vi "Automatischer Ablauf Zustandsautomat.vi"(0 "Aktion":T1) -> (2 "Aktueller test":i32, 3 "Verwendete Spangaseingänge":i32[](array[numeric]), 4 "Aktion":T1, 6 "Anzeige aktualisieren":bool, 8 "Status":string)   [LabVIEW 2020, in "EPA 1065.lvlib" / "Gas Analyzer Drift 1065-550.lvlib"]
uses:
  Gas Analyzer Drift 1065-550.lvlib
  Aktion Automatischer Ablauf Zustandsautomat.ctl
  Seiten/CalGas Aufschaltung/FGV CalGas Aktionen.ctl
  Chiller NO2 1065-376/Aktion FGV Drift Daten.ctl
  Sprachverwaltung/FGV Aktion Tabelle zerlegen.ctl
  Allgemeine VIs/Aktion Test Status.ctl
  Funktionstasten/Zustaende.ctl
  Funktionstasten/Funktionstasten-Aktion.ctl
  Seiten/CalGas Aufschaltung/Auswahl Aufschaltpunkt.ctl
  PNS/Aktionen FGV Grenzwerte.ctl
  Seiten/FT-IR/FT-IR.lvlib
  Sprachverwaltung/Sprachverwaltung.lvlib
  Seiten/CalGas Aufschaltung/CalGas Aufschaltung.lvlib
  Funktionstasten/Funktionstasten.lvlib
  PNS/PNS.lvlib
  cRIO/PC/Kommunikation mit cRIO.lvlib
  Allgemein/allgemeine Sub-VIs.lvlib
  EPA 1065.lvlib
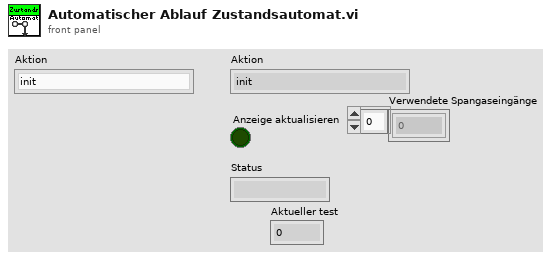
[diagram p1: front panel]
types:
  T1 = typedef "EPA 1065.lvlib/Gas Analyzer Drift 1065-550.lvlib/Aktion Automatischer Ablauf Zustandsautomat.ctl" = enum16{"init", "leerlauf", "N2 aufschalten", "N2 Aufschaltzeit warten", "N2 aufzeichnen", "CG aufschalten", "CG Aufschaltzeit warten", "CG aufzeichnen", "Span Auswahl ändern", "Test abgeschlossen", "Pre Test aktiv", "Post Test aktiv", "Störungen einlesen", "Störung", "Test anhalten", "Test fortsetzen", "Nachbehandlung init", "Nachbehandeln CG aufschalten", "Nachbehandeln CG warten", "Nachbehandeln CG aufzeichnen", "Abbrechen"}
  T2 = typedef "EPA 1065.lvlib/Aktion Test Status.ctl" = enum16{"init", "lesen", "prüfen", "Interference 366", "Interference 375", "Chiller läuft", "Drift läuft", "Pre Test läuft", "FID Optimization läuft", "FID Interference läuft"}
  T3 = typedef "EPA 1065.lvlib/Gas Analyzer Drift 1065-550.lvlib/Aktion FGV Drift Daten.ctl" = enum16{"lesen", "Konfig Daten", "PDF einstellen", "laden", "speichern", "Tabelle init", "Zeile Prüfen", "Info schreiben", "Span Einstellung", "Pre Werte schreiben", "Post Werte schreiben", "NB Pre Wert schreiben", "NB Post Wert schreiben", "Tabelle löschen"}
  T4 = typedef "Sprachverwaltung.lvlib/FGV Aktion Tabelle zerlegen.ctl" = enum16{"laden", "vereinzeln", "speichern"}
  T5 = typedef "CalGas Aufschaltung.lvlib/FGV CalGas Aktionen.ctl" = enum16{"lesen", "Analysator Auswahl", "Def.CalGas", "Aufschaltung CalGas", "laden", "speichern", "KAL extrahieren"}
  T6 = typedef "Funktionstasten.lvlib/Funktionstasten-Aktion.ctl" = enum16{"Initialisieren", "Zustand setzen", "Taste gedrückt", "Fehler speichern", "Lesen", "Manuell", "Remote", "Bitparallel", "Samplepoint", "Zeit Prüfen", "reset Umschalten"}
  T7 = typedef "Funktionstasten.lvlib/Zustaende.ctl" = enum16{"Standby", "Pause", "Eco", "Messen", "Kalibrieren", "Spülen Filter", "Spülen Leitung", "Umgebungsluft", "0-Gas", "Cal-Gas", "CG zu PNS", "-------------", "Init 1", "Init 2", "Init 3", "Init 4", "Messen vorbereiten", "Messen durchführen", "Exit"}
  T8 = typedef "CalGas Aufschaltung.lvlib/Auswahl Aufschaltpunkt.ctl" = enum16{"über Filterblock", "Analysator direkt", "über PNS", "Entnahme", "Gasdivider"}
  T9 = typedef "PNS.lvlib/Aktionen FGV Grenzwerte.ctl" = enum16{"lesen", "Grenzw. schreiben", "Anweisungscode", "IP-Adresse", "laden", "speichern", "Anweisungscode vorgeben"}
  T10 = cluster{"Pretest?":bool, "Spangaseingang":i32, "Tabellenbeginn":i32}
  T11 = cluster{"Pretest?":bool, "Spangaseingang":i32, "Tabellenbeginn":i32}[]
  T12 = typedef "CalGas Aufschaltung.lvlib/Aufschaltung CalGas.ctl" = cluster{"Kalibriergas":T13, "Aufschaltpunkt":T8, "Analysator":T14}
  T13 = typedef "Auswahlfeld.ctl" = u16
  T14 = typedef "CalGas Aufschaltung.lvlib/Auswahl Analysator.ctl" = enum16{"FT-IR", "FID", "PMA", "PMA/FID/FT-IR"}
  T15 = typedef "EPA 1065.lvlib/Gas Analyzer Drift 1065-550.lvlib/Spaninlet Cluster.ctl" = cluster{"Span Inlet Active":T16, "Analysator":T17, "Konfig Gasflasche":T16, "Gasflasche":T18, "Gasflaschen Nr.:":string, "Ablaufdatum":timestamp, "Modus":T19, "Komponenten":T20}
  T16 = typedef "System Einstellungen V2.lvlib/Konfig Gasflasche.ctl" = bool
  T17 = typedef "System Einstellungen V2.lvlib/Analysatoren.ctl" = string
  T18 = typedef "System Einstellungen V2.lvlib/Gasflasche Auswahl.ctl" = u16
  T19 = typedef "EPA 1065.lvlib/T90 Test 1065-308.lvlib/Modus.ctl" = u16
  T20 = typedef "EPA 1065.lvlib/Gas Analyzer Drift 1065-550.lvlib/Komponentencluster.ctl" = cluster{"Komponente 1":T21, "Komponente 2":T21, "Komponente 3":T21, "Komponente 4":T21, "Komponente 5":T21}
  T21 = typedef "EPA 1065.lvlib/Gas Analyzer Drift 1065-550.lvlib/Komponentenauswahl.ctl" = cluster{"Komponente:":u16, "Konzentration IST":dbl, "Einheit":enum16{"ppm", "%"}, "Genauigkeit":dbl}
  T22 = typedef "EPA 1065.lvlib/Gas Analyzer Drift 1065-550.lvlib/Konfig Daten Drift Verification.ctl" = cluster{"Bearbeiter:":string, "Pfad:":path, "Textname:":string, "CG Aufschaltzeit:":dbl, "N2 Aufschaltzeit:":dbl}
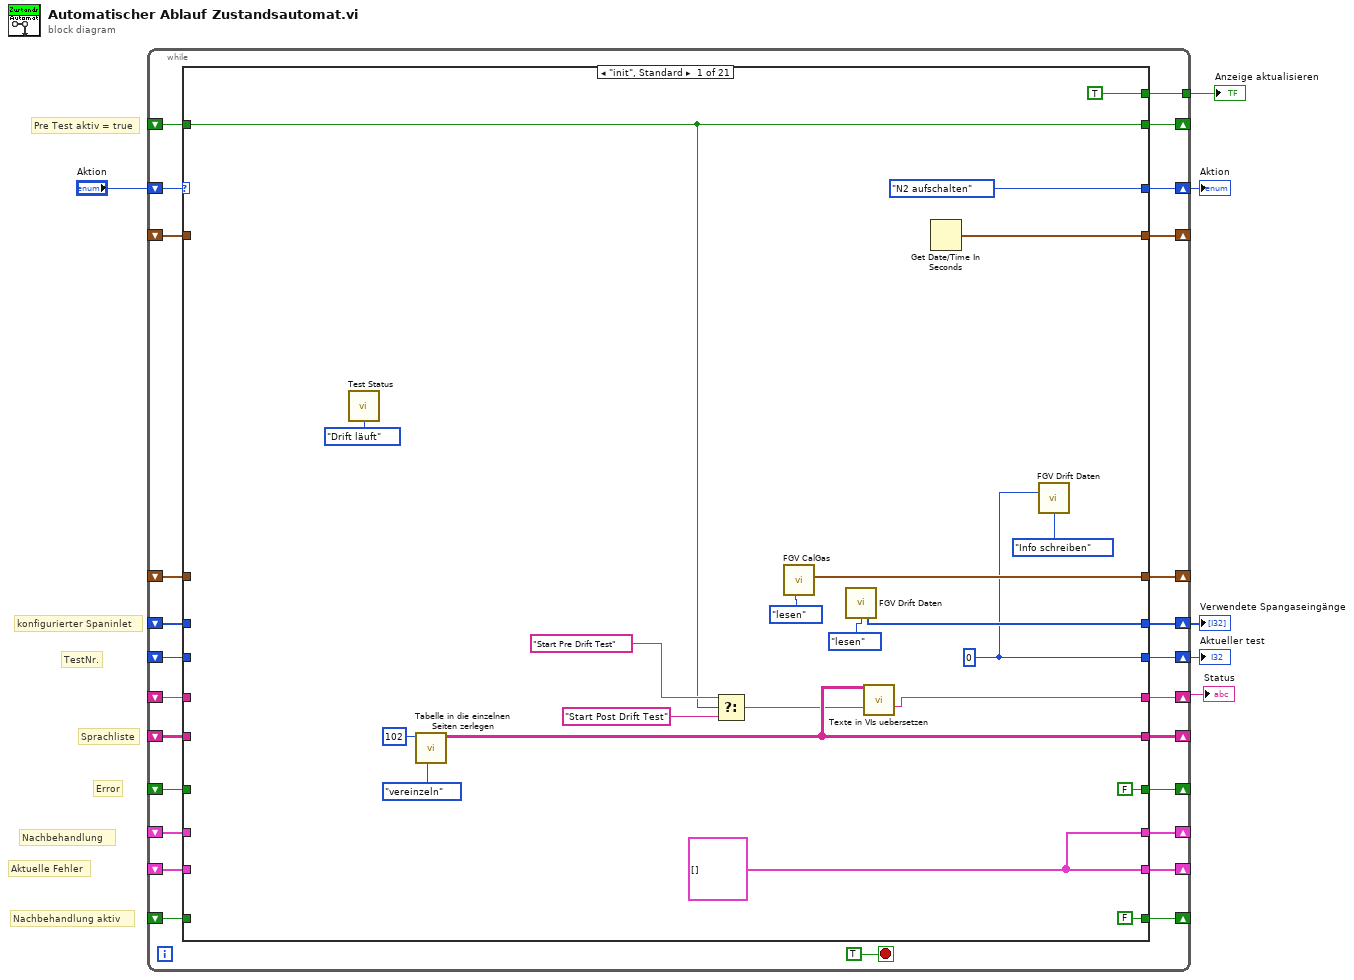
[diagram p0: block diagram]
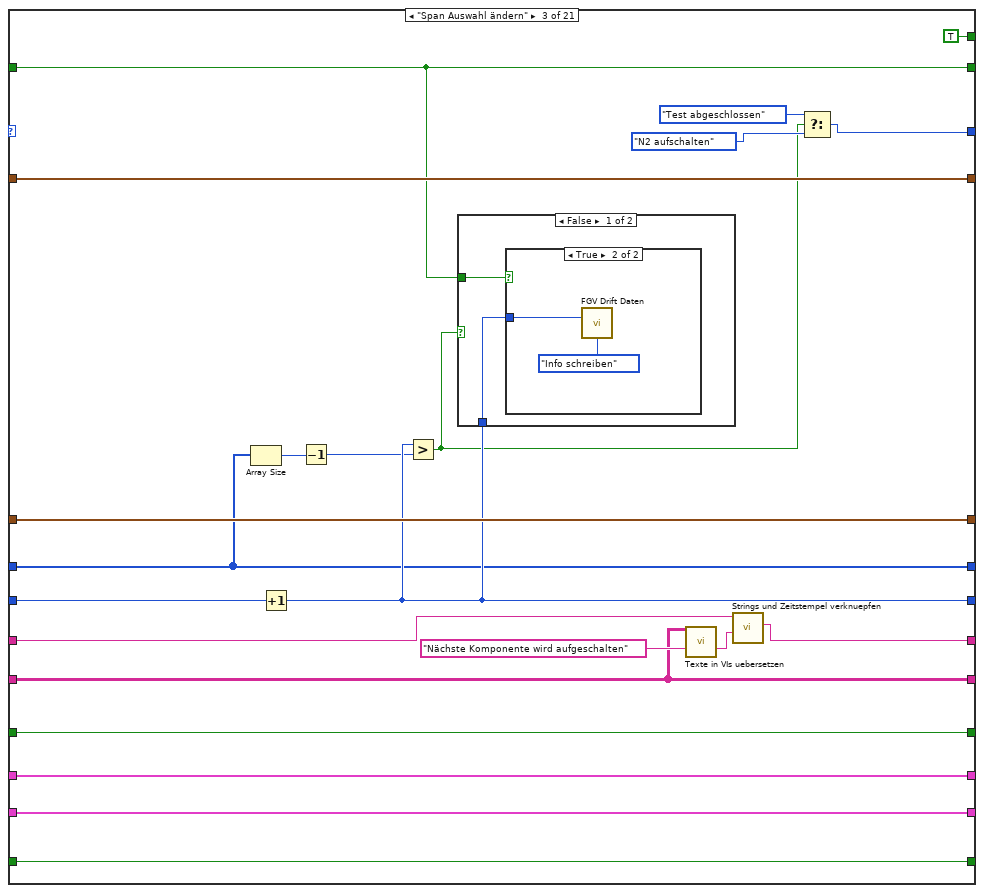
[diagram p3: hidden frame]
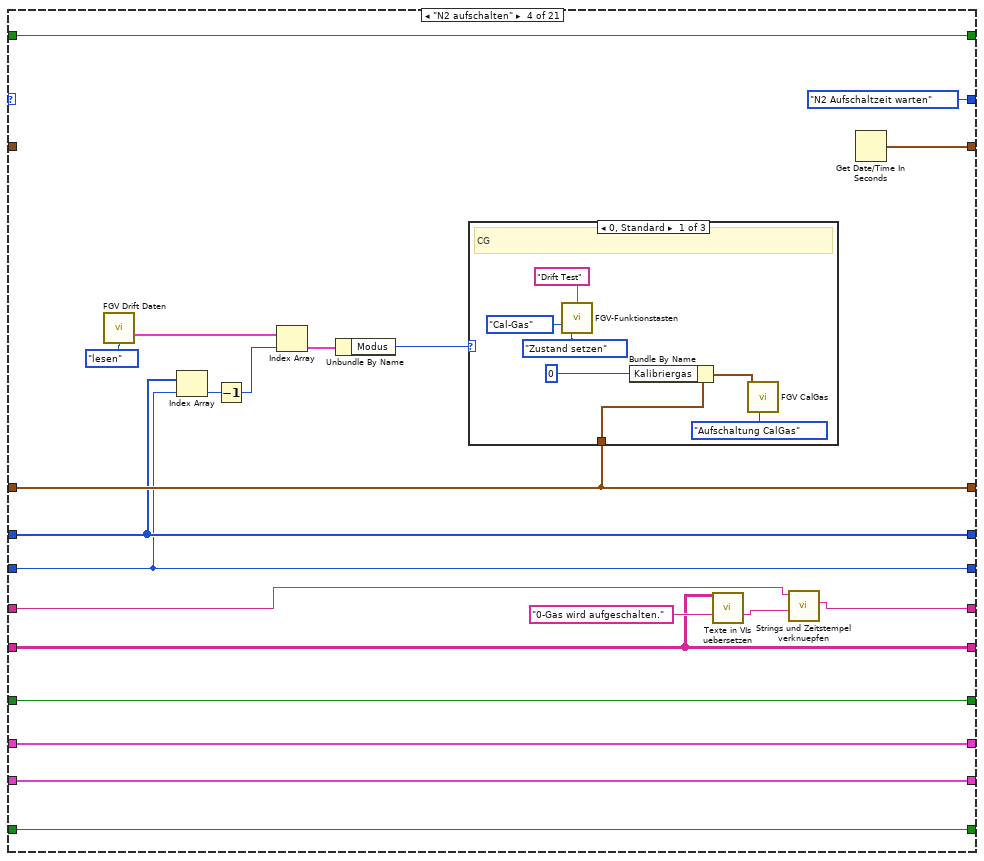
[diagram p6: hidden frame]
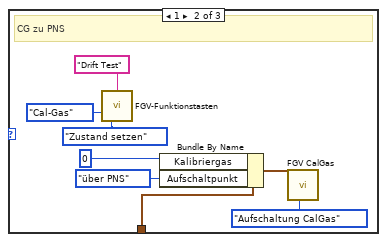
[diagram p7: hidden frame]
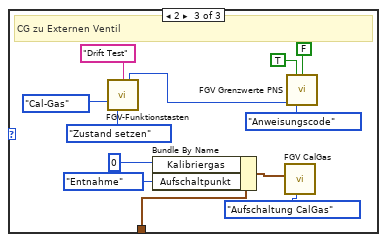
[diagram p8: hidden frame]
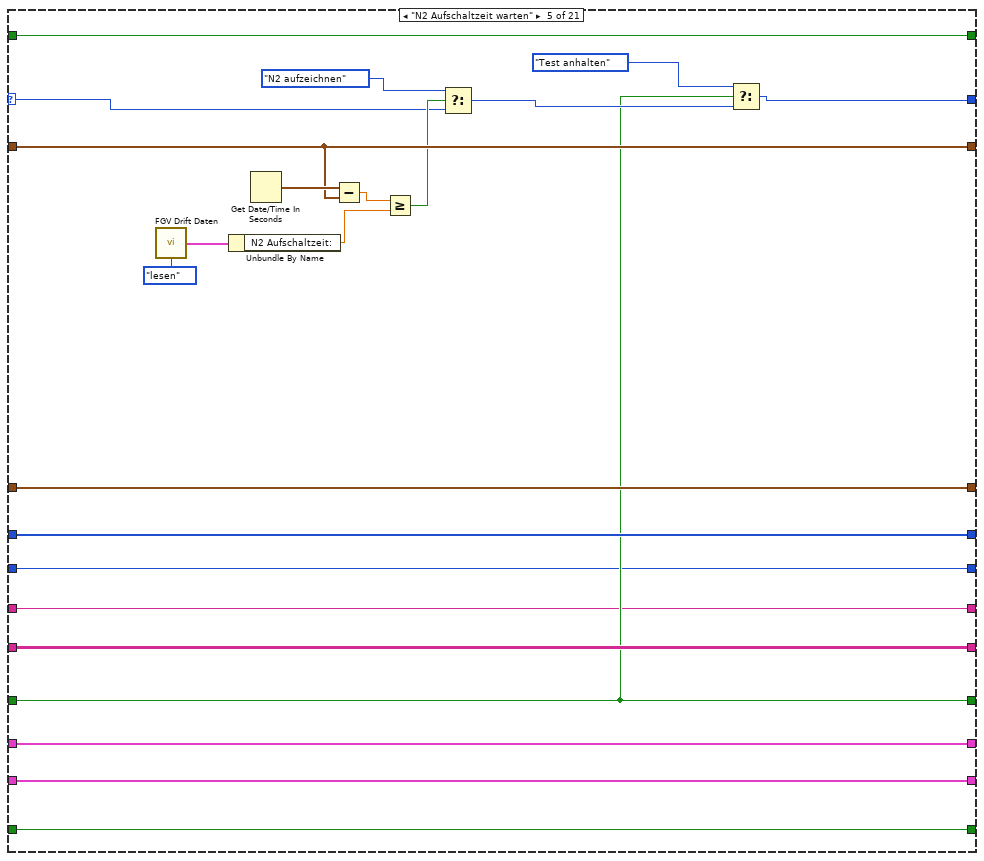
[diagram p9: hidden frame]
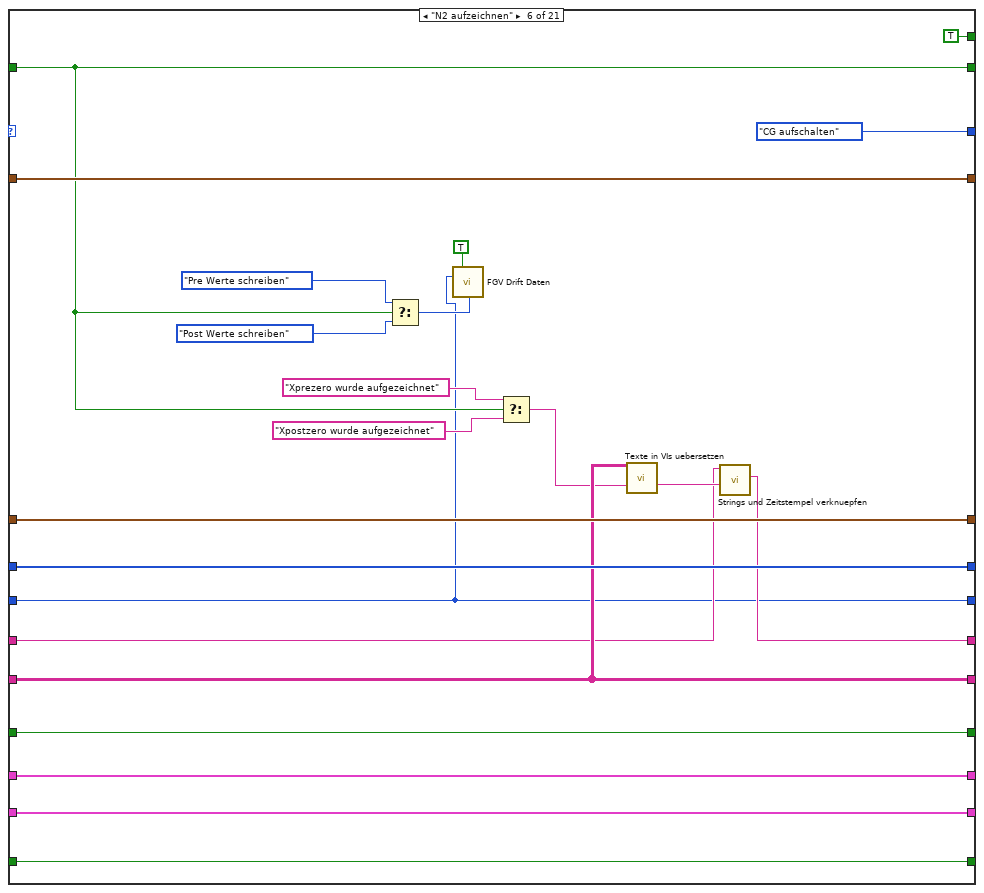
[diagram p10: hidden frame]
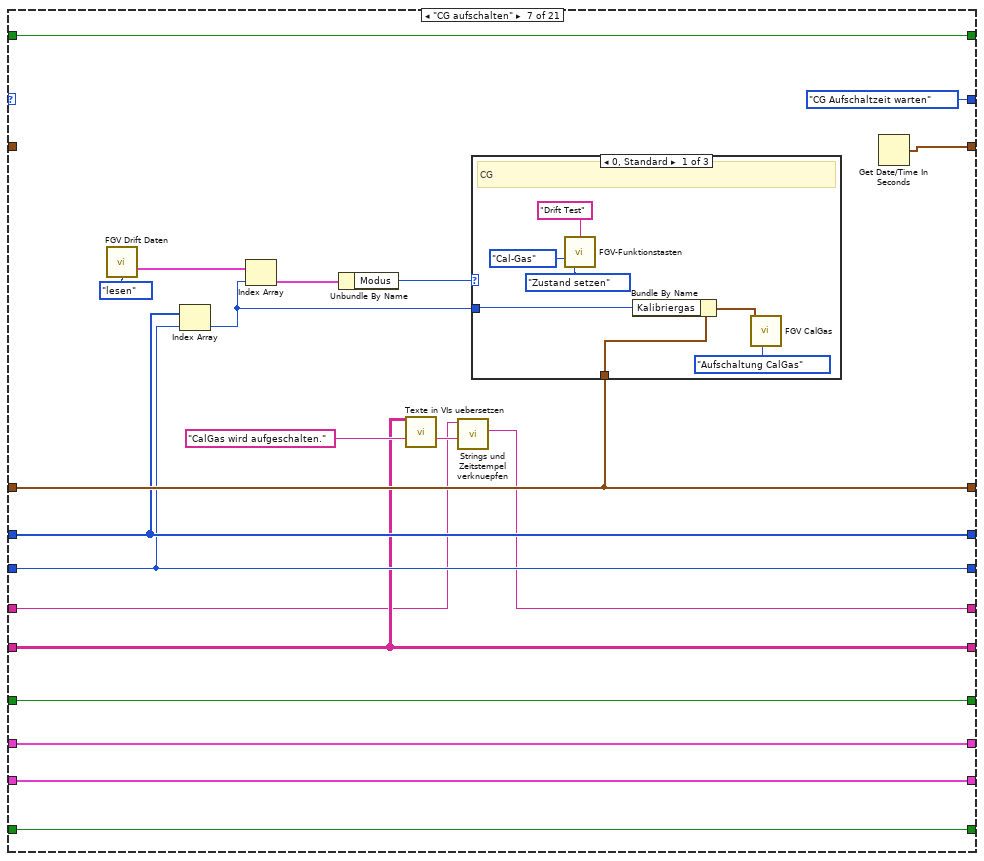
[diagram p11: hidden frame]
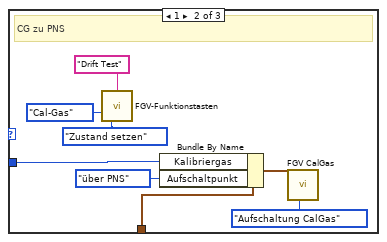
[diagram p12: hidden frame]
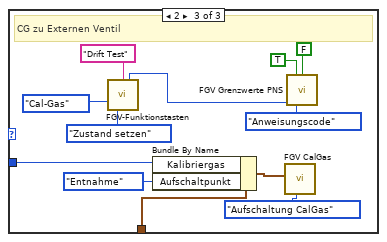
[diagram p13: hidden frame]
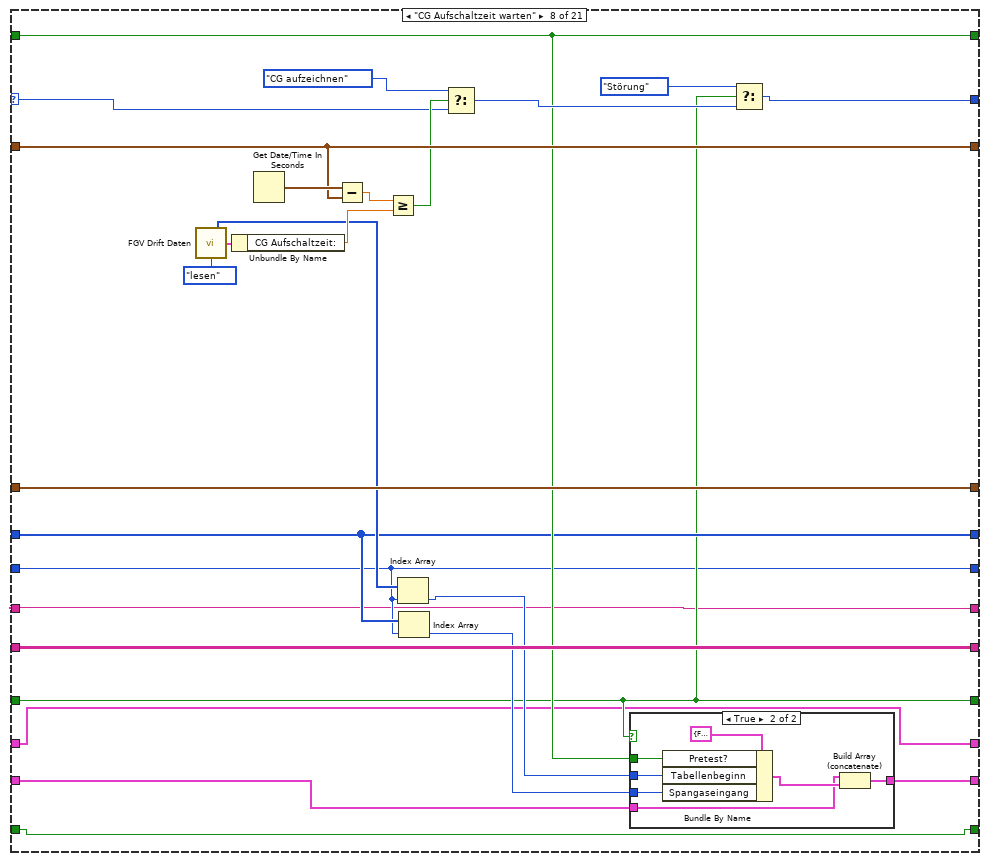
[diagram p14: hidden frame]
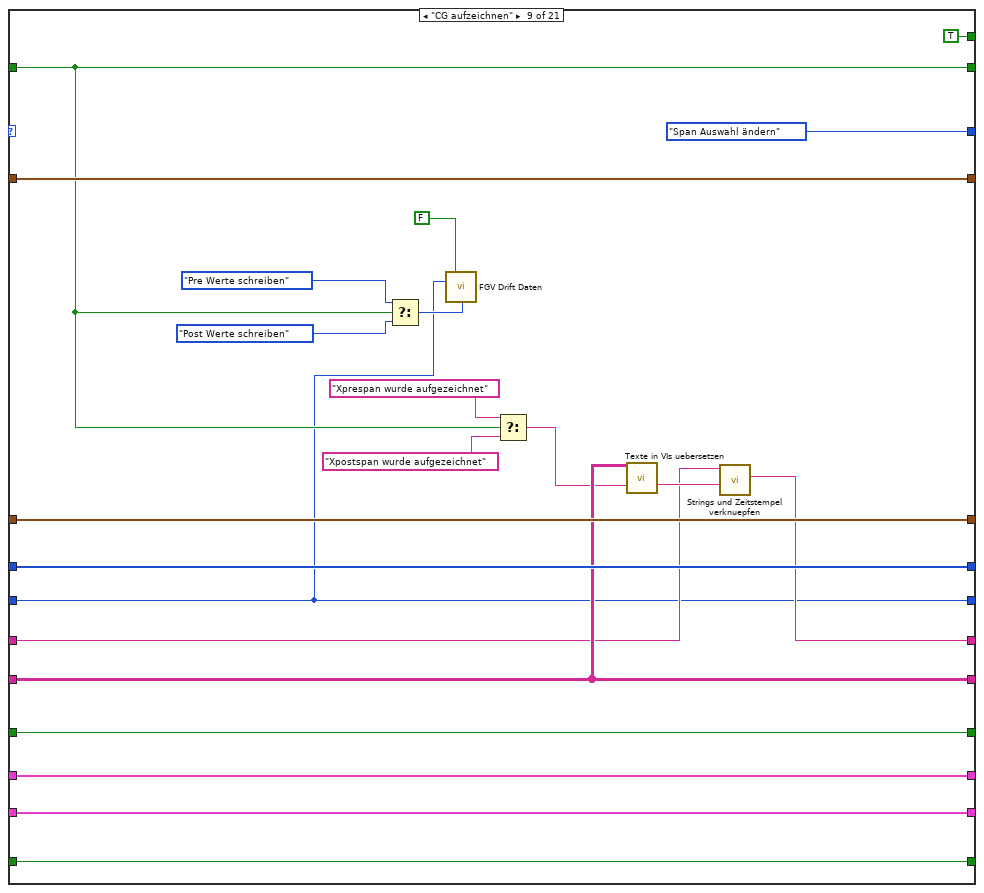
[diagram p16: hidden frame]
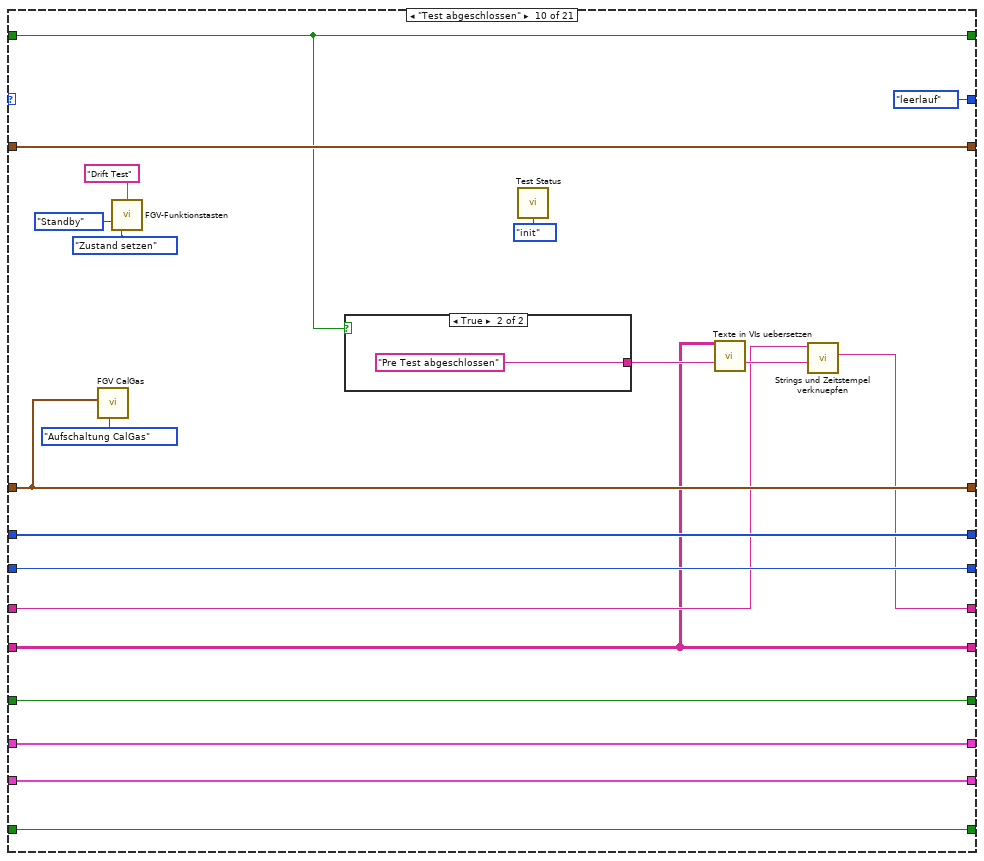
[diagram p17: hidden frame]
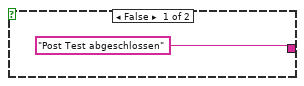
[diagram p18: hidden frame]
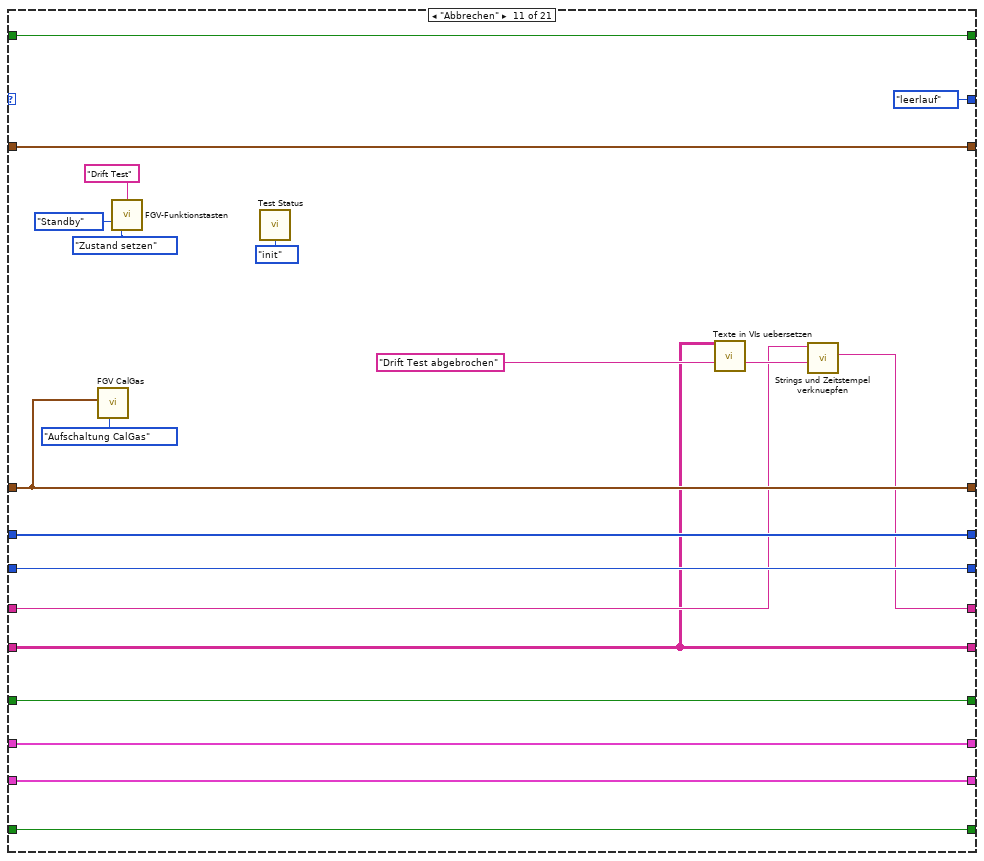
[diagram p19: hidden frame]
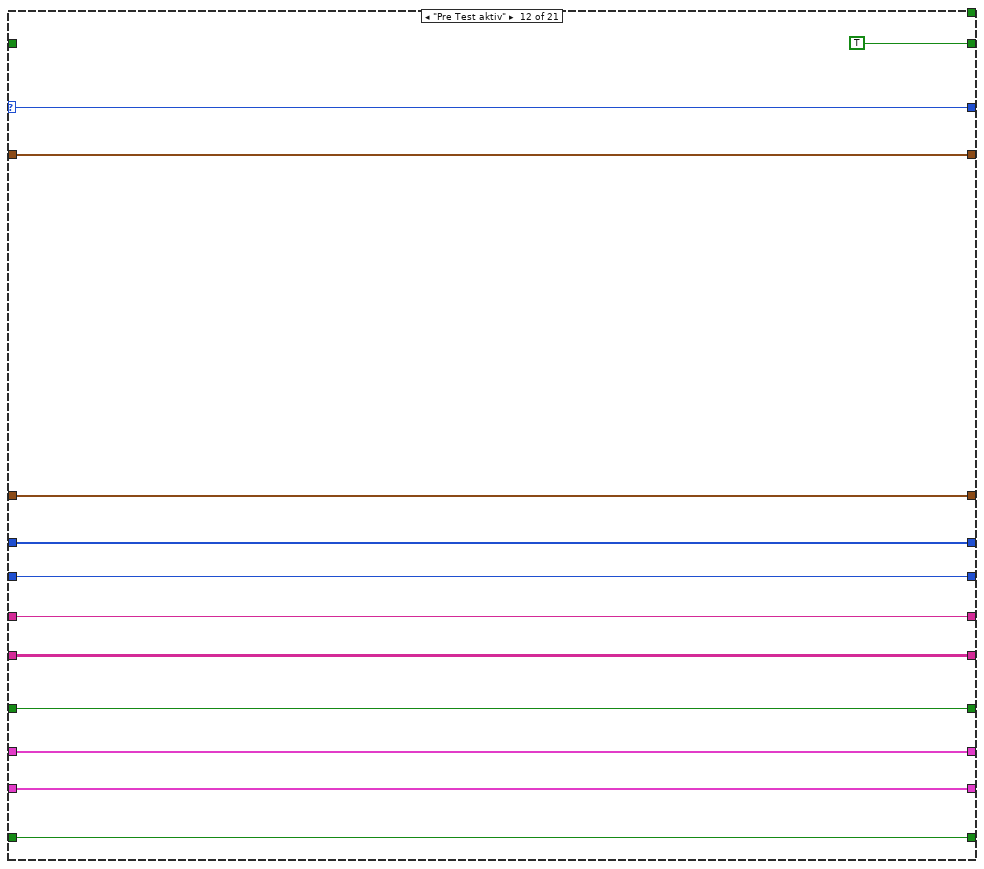
[diagram p20: hidden frame]
diagram:
  # "Nachbehandlung"
  # "Aktuelle Fehler"
  # "Nachbehandlung aktiv"
  # "TestNr."
  # "Sprachliste"
  # "Error"
  # "konfigurierter Spaninlet"
  # "Pre Test aktiv = true"
  n1 = while {
    shift-right: [w30] -> w1
    shift-left: _ -> [w29]
    shift-right: [w27] -> _
    shift-left: _ -> [w26]
    shift-right: [w25] -> _
    shift-left: _ -> [w24]
    shift-right: [w23] -> w4
    shift-left: "Aktion" -> [w31]
    shift-right: [w28] -> w2
    shift-left: _ -> [w22]
    shift-right: [w21] -> w3
    shift-left: _ -> [w20]
    shift-right: [w19] -> _
    shift-left: _ -> [w18]
    shift-right: [w17] -> _
    shift-left: _ -> [w16]
    shift-right: [w15] -> _
    shift-left: _ -> [w14]
    shift-right: [w13] -> _
    shift-left: _ -> [w12]
    shift-right: [w11] -> _
    shift-left: _ -> [w10]
    shift-right: [w9] -> _
    shift-left: _ -> [w8]
    tunnel: [w7] -> w5
    stop <- TRUE stop-if-true
    n2 = case shown="\"init\", Standard" w31 {
      selector: w31 -> [_ w54 _ _ w153 _ _ w248 _ _ _ w336 w349 w360 _ _ _ _ _ w507 _]
      tunnel: [w39 w59 w67 w94 w140 w175 w188 w231 w276 w289 w311 w334 w341 w358 w380 w402 w416 w427 w451 w492 w531] -> w30
      tunnel: w29 -> [_ w59 w68 w95 w140 w176 w189 w231 w277 w291 w313 w334 w341 w358 w381 w403 w417 w428 w452 w492 w532]
      tunnel: [w44 w57 w82 w106 w143 w167 w197 w234 w269 w302 w324 w335 w344 w359 w386 w400 w415 0 w449 w494 w523] -> w28
      tunnel: [w34 w65 w83 w112 w147 w173 w203 w242 w274 w288 w310 TRUE FALSE w377 w392 w411 w426 w431 w446 w501 w529] -> w27
      tunnel: w26 -> [w34 w65 w83 w112 w147 w173 w203 w242 w274 w288 w310 _ _ w377 w392 w411 w426 w431 _ w501 w529]
      tunnel: [w52 w64 w87 w111 w161 w183 w202 w256 w286 w299 w321 w339 w351 w376 w391 w394 w425 w436 w464 w515 w541] -> w25
      tunnel: w24 -> [_ w64 w87 w111 w161 w183 w202 w256 w286 w299 w321 w339 w351 w376 w391 w394 w425 w436 w464 w515 w541]
      tunnel: [Aktion_Automatischer_Ablauf_Zustandsautomat."N2 aufschalten" ("Aktion") w54 w77 Aktion_Automatischer_Ablauf_Zustandsautomat."N2 Aufschaltzeit warten" ("Aktion") w148 Aktion_Automatischer_Ablauf_Zustandsautomat."CG aufschalten" ("Aktion") Aktion_Automatischer_Ablauf_Zustandsautomat."CG Aufschaltzeit warten" ("Aktion") w243 Aktion_Automatischer_Ablauf_Zustandsautomat."Span Auswahl ändern" ("Aktion") Aktion_Automatischer_Ablauf_Zustandsautomat."leerlauf" ("Aktion") Aktion_Automatischer_Ablauf_Zustandsautomat."leerlauf" ("Aktion") w336 w349 w360 Aktion_Automatischer_Ablauf_Zustandsautomat."Span Auswahl ändern" ("Aktion") Aktion_Automatischer_Ablauf_Zustandsautomat."leerlauf" ("Aktion") Aktion_Automatischer_Ablauf_Zustandsautomat."N2 aufschalten" ("Aktion") Aktion_Automatischer_Ablauf_Zustandsautomat."Nachbehandeln CG aufschalten" ("Aktion") Aktion_Automatischer_Ablauf_Zustandsautomat."Nachbehandeln CG warten" ("Aktion") w502 Aktion_Automatischer_Ablauf_Zustandsautomat."Span Auswahl ändern" ("Aktion")] -> w23
      tunnel: w22 -> [_ w57 w84 w106 w143 w167 w197 w234 w269 w302 w324 w335 w344 w359 w386 w400 w415 _ w449 w494 w523]
      tunnel: [w49 w63 w81 w107 w146 w182 w198 w240 w285 w306 w328 w338 w350 w375 w390 w410 w424 w438 w460 w500 w540] -> w21
      tunnel: w20 -> [_ w63 w81 w107 w146 w182 w198 w240 w285 w306 w328 w338 w350 w375 w390 w410 w424 w438 w460 w500 w540]
      tunnel: [FALSE w62 w86 w103 w145 w181 w194 w235 w284 w305 w327 w337 w348 w362 w389 w409 w423 FALSE w458 w497 w539] -> w19
      tunnel: w18 -> [_ w62 w86 w103 w145 w181 w194 w235 w284 w305 w327 w337 w348 _ w389 w409 w423 _ w458 w497 w539]
      tunnel: [w47 w61 w85 w99 w155 w180 w184 w250 w283 w304 w326 w333 w347 w357 w388 w408 w422 w441 w457 w509 w538] -> w17
      tunnel: w16 -> [_ w61 w85 _ w155 w180 _ w250 w283 w304 w326 w333 w347 w357 w388 w408 w422 _ w457 w509 w538]
      tunnel: [w40 w60 w69 w96 w151 w178 w190 w246 w279 w290 w312 w332 w346 w356 w378 w404 w418 w430 w453 w505 w534] -> w15
      tunnel: w14 -> [_ w60 w69 w96 w151 w178 w190 w246 w279 w290 w312 w332 w346 w356 w378 w404 w418 w430 w453 w505 w534]
      tunnel: [w41 w58 w74 w102 w144 w165 w187 w237 w268 w303 w325 w331 w345 w355 w387 w407 w421 w439 w448 w499 w522] -> w13
      tunnel: w12 -> [_ w58 w74 w102 w144 w165 w187 w236 w268 w303 w325 w331 w345 w355 w387 w407 w421 w439 w448 w498 w522]
      tunnel: [FALSE w56 w73 w101 w142 w164 w186 w233 w267 w301 w323 w330 w343 w354 w385 w396 w413 TRUE w450 w496 w524] -> w11
      tunnel: w10 -> [_ w56 w73 w101 w142 w164 w186 w233 w267 w301 w323 w330 w343 w354 w385 w396 w413 _ w450 w496 w524]
      tunnel: [w41 w55 w72 w100 w141 w163 w185 w232 w266 w294 w316 w329 w342 w353 w384 w393 w412 w435 w444 w495 w521] -> w9
      tunnel: w8 -> [_ w55 w72 w100 w141 w163 w185 w232 w266 w294 w316 w329 w342 w353 w384 w393 w412 w435 w444 w495 w521]
      tunnel: [TRUE _ TRUE _ _ TRUE _ _ TRUE _ _ _ _ _ _ _ _ _ _ _ TRUE] -> w7
      frame "init", Default {
        w41 = T11 []
        w44 = 0
        n3 = call "Test Status.vi"("Aktion"=Aktion_Test_Status."Drift läuft") -> ()  [unwired: 11 in, 4 out]
        n4 = call "Tabelle in die einzelnen Seiten zerlegen.vi"("Aktion"=FGV_Aktion_Tabelle_zerlegen."vereinzeln", "Index (Seite)"=102) -> ("Sprachliste"=w40:string[][])  [unwired: 7 in, 2 out]
        n5 = Select(t="Start Pre Drift Test", s=w34, f="Start Post Drift Test") -> (s? t:f=w33:string)
        n6 = call "FGV CalGas.vi"("Aktionen"=FGV_CalGas_Aktionen."lesen") -> ("Aufschaltung CalGas"=w52:T12)  [unwired: 6 in, 4 out]
        n7 = call "FGV Drift Daten.vi"("Aktion"=Aktion_FGV_Drift_Daten."lesen") -> ("Verwendete Spangaseingänge"=w49:i32[])  [unwired: 7 in, 7 out]
        n8 = call "Texte in VIs uebersetzen.vi"("Sprachliste"=w40, "String zum Übersetzen"=w33) -> ("String zum Übersetzen"=w39:string)  [unwired: 9 in, 4 out]
        n9 = Get Date/Time In Seconds() -> (seconds since 1Jan1904=w47:timestamp)
        n10 = call "FGV Drift Daten.vi"("Testnr."=w44, "Aktion"=Aktion_FGV_Drift_Daten."Info schreiben") -> ()  [unwired: 6 in, 8 out]
      }
      frame "leerlauf" {
      }
      frame "Span Auswahl ändern" {
        n11 = Array Size(array=w81) -> (size(s)=w80:i32)
        n12 = Increment(x=w84) -> (x+1=w82:i32)
        n13 = Decrement(x=w80) -> (x-1=w79:i32)
        n14 = Greater?(x=w82, y=w79) -> (0:w75:bool)
        n15 = case shown="False" w75 {
          tunnel: w83 -> [w89 _]
          tunnel: w82 -> [w88 _]
          frame False {
            n16 = case shown="True" w89 {
              tunnel: w88 -> [_ w90]
              frame False {
              }
              frame True {
                n17 = call "FGV Drift Daten.vi"("Testnr."=w90, "Aktion"=Aktion_FGV_Drift_Daten."Info schreiben") -> ()  [unwired: 6 in, 8 out]
              }
            }
          }
          frame True {
          }
        }
        n18 = call "Texte in VIs uebersetzen.vi"("Sprachliste"=w69, "String zum Übersetzen"="Nächste Komponente wird aufgeschalten" ("String 1 hinzufügen")) -> ("String zum Übersetzen"=w71:string)  [unwired: 9 in, 4 out]
        n19 = call "Strings und Zeitstempel verknuepfen.vi"("String 1 hinzufügen"=w71, "Eingagns String"=w68) -> ("Verknüpfter String"=w67:string)  [unwired: 9 in]
        n20 = Select(t=Aktion_Automatischer_Ablauf_Zustandsautomat."Test abgeschlossen", s=w75, f=Aktion_Automatischer_Ablauf_Zustandsautomat."N2 aufschalten" ("Aktion")) -> (s? t:f=w77:T1)
      }
      frame "N2 aufschalten" {
        n21 = call "FGV Drift Daten.vi"("Aktion"=Aktion_FGV_Drift_Daten."lesen") -> ("Spangaseinstellungen"=w109:T15[])  [unwired: 7 in, 7 out]
        n22 = Index Array(array=w107, index=w106) -> (element=w105:i32)
        n23 = Decrement(x=w105) -> (x-1=w92:i32)
        n24 = Index Array(array=w109, index=w92) -> (element=w108:T15)
        n25 = Unbundle By Name(w108) -> ("Modus"=w104:T19)
        n26 = case shown="0, Standard" w104 {
          tunnel: w111 -> [w114 w121 w129]
          frame 0, Default {
            # "CG"
            n27 = call "FGV-Funktionstasten.vi"("Herkunft"="Drift Test", "Zustand"=Zustaende."Cal-Gas", "Aktion"=Funktionstasten-Aktion."Zustand setzen") -> ()  [unwired: 5 in, 8 out]
            n28 = Bundle By Name(cluster=w114, "Kalibriergas"=u16 0) -> (w115:T12)
            n29 = call "FGV CalGas.vi"("Aktionen"=FGV_CalGas_Aktionen."Aufschaltung CalGas", "Aufschaltung CalGas"=w115) -> ()  [unwired: 5 in, 5 out]
          }
          frame 1 {
            # "CG zu PNS"
            n30 = call "FGV-Funktionstasten.vi"("Herkunft"="Drift Test", "Zustand"=Zustaende."Cal-Gas", "Aktion"=Funktionstasten-Aktion."Zustand setzen") -> ()  [unwired: 5 in, 8 out]
            n31 = Bundle By Name(cluster=w121, "Kalibriergas"=u16 0, "Aufschaltpunkt"=Auswahl_Aufschaltpunkt."über PNS") -> (w122:T12)
            n32 = call "FGV CalGas.vi"("Aktionen"=FGV_CalGas_Aktionen."Aufschaltung CalGas", "Aufschaltung CalGas"=w122) -> ()  [unwired: 5 in, 5 out]
          }
          frame 2 {
            # "CG zu Externen Ventil"
            n33 = call "FGV-Funktionstasten.vi"("Herkunft"="Drift Test", "Zustand"=Zustaende."Cal-Gas", "Aktion"=Funktionstasten-Aktion."Zustand setzen") -> ("Samplepoint"=w133:u16)  [unwired: 5 in, 7 out]
            n34 = Bundle By Name(cluster=w129, "Kalibriergas"=u16 0, "Aufschaltpunkt"=Auswahl_Aufschaltpunkt."Entnahme") -> (w130:T12)
            n35 = call "FGV CalGas.vi"("Aktionen"=FGV_CalGas_Aktionen."Aufschaltung CalGas", "Aufschaltung CalGas"=w130) -> ()  [unwired: 5 in, 5 out]
            n36 = call "FGV Grenzwerte PNS.vi"("T90"=TRUE ("T90 lüften"), "T90 lüften"=FALSE, "Samplepoint"=w133, "Aktionen FGV Grenzwerte"=Aktionen_FGV_Grenzwerte."Anweisungscode") -> ()  [unwired: 9 in, 3 out]
          }
        }
        n37 = call "Texte in VIs uebersetzen.vi"("Sprachliste"=w96, "String zum Übersetzen"="0-Gas wird aufgeschalten." ("String 1 hinzufügen")) -> ("String zum Übersetzen"=w93:string)  [unwired: 9 in, 4 out]
        n38 = call "Strings und Zeitstempel verknuepfen.vi"("String 1 hinzufügen"=w93, "Eingagns String"=w95) -> ("Verknüpfter String"=w94:string)  [unwired: 9 in]
        n39 = Get Date/Time In Seconds() -> (seconds since 1Jan1904=w99:timestamp)
      }
      frame "N2 Aufschaltzeit warten" {
        n40 = call "FGV Drift Daten.vi"("Aktion"=Aktion_FGV_Drift_Daten."lesen") -> ("Drift Konfig Daten"=w159:T22)  [unwired: 7 in, 7 out]
        n41 = Unbundle By Name(w159) -> ("N2 Aufschaltzeit:"=w157:dbl)
        n42 = Get Date/Time In Seconds() -> (seconds since 1Jan1904=w160:timestamp)
        n43 = Subtract(x=w160, y=w155) -> (x-y=w158:dbl)
        n44 = Greater Or Equal?(x=w158, y=w157) -> (x >= y?=w154:bool)
        n45 = Select(t=Aktion_Automatischer_Ablauf_Zustandsautomat."N2 aufzeichnen", s=w154, f=w153) -> (s? t:f=w149:T1)
        n46 = Select(t=Aktion_Automatischer_Ablauf_Zustandsautomat."Test anhalten", s=w145, f=w149) -> (s? t:f=w148:T1)
      }
      frame "N2 aufzeichnen" {
        n47 = Select(t=Aktion_FGV_Drift_Daten."Pre Werte schreiben" ("Aktion"), s=w173, f=Aktion_FGV_Drift_Daten."Post Werte schreiben" ("Aktion")) -> (s? t:f=w171:T3)
        n48 = call "FGV Drift Daten.vi"("0-Gas Wert?"=TRUE, "Testnr."=w167, "Aktion"=w171) -> ()  [unwired: 5 in, 8 out]
        n49 = Select(t="Xprezero wurde aufgezeichnet" ("String 1 hinzufügen"), s=w173, f="Xpostzero wurde aufgezeichnet" ("String 1 hinzufügen")) -> (s? t:f=w177:string)
        n50 = call "Texte in VIs uebersetzen.vi"("Sprachliste"=w178, "String zum Übersetzen"=w177) -> ("String zum Übersetzen"=w179:string)  [unwired: 9 in, 4 out]
        n51 = call "Strings und Zeitstempel verknuepfen.vi"("String 1 hinzufügen"=w179, "Eingagns String"=w176) -> ("Verknüpfter String"=w175:string)  [unwired: 9 in]
      }
      frame "CG aufschalten" {
        n52 = call "FGV Drift Daten.vi"("Aktion"=Aktion_FGV_Drift_Daten."lesen") -> ("Spangaseinstellungen"=w200:T15[])  [unwired: 7 in, 7 out]
        n53 = Index Array(array=w198, index=w197) -> (element=w195:i32)
        n54 = Index Array(array=w200, index=w195) -> (element=w199:T15)
        n55 = Unbundle By Name(w199) -> ("Modus"=w196:T19)
        n56 = call "Texte in VIs uebersetzen.vi"("Sprachliste"=w190, "String zum Übersetzen"="CalGas wird aufgeschalten." ("String 1 hinzufügen")) -> ("String zum Übersetzen"=w192:string)  [unwired: 9 in, 4 out]
        n57 = call "Strings und Zeitstempel verknuepfen.vi"("String 1 hinzufügen"=w192, "Eingagns String"=w189) -> ("Verknüpfter String"=w188:string)  [unwired: 9 in]
        n58 = case shown="0, Standard" w196 {
          tunnel: w202 -> [w205 w212 w220]
          tunnel: w195 -> [w204 w211 w219]
          frame 0, Default {
            # "CG"
            n59 = call "FGV-Funktionstasten.vi"("Herkunft"="Drift Test", "Zustand"=Zustaende."Cal-Gas", "Aktion"=Funktionstasten-Aktion."Zustand setzen") -> ()  [unwired: 5 in, 8 out]
            n60 = Bundle By Name(cluster=w205, "Kalibriergas"=w204) -> (w206:T12)
            n61 = call "FGV CalGas.vi"("Aktionen"=FGV_CalGas_Aktionen."Aufschaltung CalGas", "Aufschaltung CalGas"=w206) -> ()  [unwired: 5 in, 5 out]
          }
          frame 1 {
            # "CG zu PNS"
            n62 = call "FGV-Funktionstasten.vi"("Herkunft"="Drift Test", "Zustand"=Zustaende."Cal-Gas", "Aktion"=Funktionstasten-Aktion."Zustand setzen") -> ()  [unwired: 5 in, 8 out]
            n63 = Bundle By Name(cluster=w212, "Kalibriergas"=w211, "Aufschaltpunkt"=Auswahl_Aufschaltpunkt."über PNS") -> (w213:T12)
            n64 = call "FGV CalGas.vi"("Aktionen"=FGV_CalGas_Aktionen."Aufschaltung CalGas", "Aufschaltung CalGas"=w213) -> ()  [unwired: 5 in, 5 out]
          }
          frame 2 {
            # "CG zu Externen Ventil"
            n65 = call "FGV-Funktionstasten.vi"("Herkunft"="Drift Test", "Zustand"=Zustaende."Cal-Gas", "Aktion"=Funktionstasten-Aktion."Zustand setzen") -> ("Samplepoint"=w224:u16)  [unwired: 5 in, 7 out]
            n66 = Bundle By Name(cluster=w220, "Kalibriergas"=w219, "Aufschaltpunkt"=Auswahl_Aufschaltpunkt."Entnahme") -> (w221:T12)
            n67 = call "FGV CalGas.vi"("Aktionen"=FGV_CalGas_Aktionen."Aufschaltung CalGas", "Aufschaltung CalGas"=w221) -> ()  [unwired: 5 in, 5 out]
            n68 = call "FGV Grenzwerte PNS.vi"("T90"=TRUE ("T90 lüften"), "T90 lüften"=FALSE, "Samplepoint"=w224, "Aktionen FGV Grenzwerte"=Aktionen_FGV_Grenzwerte."Anweisungscode") -> ()  [unwired: 9 in, 3 out]
          }
        }
        n69 = Get Date/Time In Seconds() -> (seconds since 1Jan1904=w184:timestamp)
      }
      frame "CG Aufschaltzeit warten" {
        n70 = call "FGV Drift Daten.vi"("Aktion"=Aktion_FGV_Drift_Daten."lesen") -> ("Tabellenbeginn"=w241:i32[], "Drift Konfig Daten"=w254:T22)  [unwired: 7 in, 6 out]
        n71 = Unbundle By Name(w254) -> ("CG Aufschaltzeit:"=w252:dbl)
        n72 = Get Date/Time In Seconds() -> (seconds since 1Jan1904=w255:timestamp)
        n73 = Subtract(x=w255, y=w250) -> (x-y=w253:dbl)
        n74 = Greater Or Equal?(x=w253, y=w252) -> (x >= y?=w249:bool)
        n75 = Index Array(array=w241, index=w234) -> (element=w239:i32)
        n76 = Index Array(array=w240, index=w234) -> (element=w238:i32)
        n77 = Select(t=Aktion_Automatischer_Ablauf_Zustandsautomat."CG aufzeichnen", s=w249, f=w248) -> (s? t:f=w244:T1)
        n78 = case shown="True" w235 {
          tunnel: w242 -> [_ w264]
          tunnel: w239 -> [_ w262]
          tunnel: w238 -> [_ w261]
          tunnel: [w257 w259] -> w237
          tunnel: w236 -> [w257 w258]
          frame False {
          }
          frame True {
            n79 = Bundle By Name(cluster=T10 {"Pretest?"=FALSE, "Spangaseingang"=0, "Tabellenbeginn"=0} ("Eingangs-Cluster"), "Pretest?"=w264, "Tabellenbeginn"=w262, "Spangaseingang"=w261) -> (w260:T10)
            n80 = Build Array (concatenate)(w258, w260) -> (w259:T11)
          }
        }
        n81 = Select(t=Aktion_Automatischer_Ablauf_Zustandsautomat."Störung", s=w235, f=w244) -> (s? t:f=w243:T1)
      }
      frame "CG aufzeichnen" {
        n82 = Select(t=Aktion_FGV_Drift_Daten."Pre Werte schreiben" ("Aktion"), s=w274, f=Aktion_FGV_Drift_Daten."Post Werte schreiben" ("Aktion")) -> (s? t:f=w272:T3)
        n83 = call "FGV Drift Daten.vi"("0-Gas Wert?"=FALSE, "Testnr."=w269, "Aktion"=w272) -> ()  [unwired: 5 in, 8 out]
        n84 = Select(t="Xprespan wurde aufgezeichnet" ("String 1 hinzufügen"), s=w274, f="Xpostspan wurde aufgezeichnet" ("String 1 hinzufügen")) -> (s? t:f=w278:string)
        n85 = call "Texte in VIs uebersetzen.vi"("Sprachliste"=w279, "String zum Übersetzen"=w278) -> ("String zum Übersetzen"=w280:string)  [unwired: 9 in, 4 out]
        n86 = call "Strings und Zeitstempel verknuepfen.vi"("String 1 hinzufügen"=w280, "Eingagns String"=w277) -> ("Verknüpfter String"=w276:string)  [unwired: 9 in]
      }
      frame "Test abgeschlossen" {
        n87 = call "FGV CalGas.vi"("Aktionen"=FGV_CalGas_Aktionen."Aufschaltung CalGas", "Aufschaltung CalGas"=w299) -> ()  [unwired: 5 in, 5 out]
        n88 = call "FGV-Funktionstasten.vi"("Herkunft"="Drift Test", "Zustand"=Zustaende."Standby", "Aktion"=Funktionstasten-Aktion."Zustand setzen") -> ()  [unwired: 5 in, 8 out]
        n89 = case shown="True" w288 {
          tunnel: ["Post Test abgeschlossen" ("String zum Übersetzen") "Pre Test abgeschlossen" ("String zum Übersetzen")] -> w292
          frame False {
          }
          frame True {
          }
        }
        n90 = call "Test Status.vi"("Aktion"=Aktion_Test_Status."init") -> ()  [unwired: 11 in, 4 out]
        n91 = call "Texte in VIs uebersetzen.vi"("Sprachliste"=w290, "String zum Übersetzen"=w292) -> ("String zum Übersetzen"=w293:string)  [unwired: 9 in, 4 out]
        n92 = call "Strings und Zeitstempel verknuepfen.vi"("String 1 hinzufügen"=w293, "Eingagns String"=w291) -> ("Verknüpfter String"=w289:string)  [unwired: 9 in]
      }
      frame "Abbrechen" {
        n93 = call "FGV CalGas.vi"("Aktionen"=FGV_CalGas_Aktionen."Aufschaltung CalGas", "Aufschaltung CalGas"=w321) -> ()  [unwired: 5 in, 5 out]
        n94 = call "FGV-Funktionstasten.vi"("Herkunft"="Drift Test", "Zustand"=Zustaende."Standby", "Aktion"=Funktionstasten-Aktion."Zustand setzen") -> ()  [unwired: 5 in, 8 out]
        n95 = call "Test Status.vi"("Aktion"=Aktion_Test_Status."init") -> ()  [unwired: 11 in, 4 out]
        n96 = call "Texte in VIs uebersetzen.vi"("Sprachliste"=w312, "String zum Übersetzen"="Drift Test abgebrochen") -> ("String zum Übersetzen"=w315:string)  [unwired: 9 in, 4 out]
        n97 = call "Strings und Zeitstempel verknuepfen.vi"("String 1 hinzufügen"=w315, "Eingagns String"=w313) -> ("Verknüpfter String"=w311:string)  [unwired: 9 in]
      }
      frame "Pre Test aktiv" {
      }
      frame "Post Test aktiv" {
      }
      frame "Störungen einlesen" {
        # "Druck CG"
        # "Durchfluss FTIR ab min"
        n98 = call "FGV cRIO-Daten.vi"("Aktion"=enum16{"lesen", "schreiben"}."lesen") -> ("Störungen"=w374:u64[])  [unwired: 9 in, 9 out]
        n99 = Index Array(array=w374, index=0 ("Index")) -> (element=w372:u64)
        n100 = Number To Boolean Array(number=w372) -> (Boolean array=w370:bool[])
        n101 = Index Array(array=w370, index #1=95 ("Index"), index #2=68 ("Index")) -> (element #1=w368:bool, element #2=w361:bool)
        n102 = call "Verzoegerung PC.vi"("sec"=u16 5, "Startsignal"=w368) -> ("Zeit abgelaufen?"=w363:bool)  [unwired: 8 in, 1 out]
        n103 = call "Verzoegerung PC.vi"("sec"=u16 5, "Startsignal"=w361) -> ("Zeit abgelaufen?"=w364:bool)  [unwired: 8 in, 1 out]
        n104 = And(x=w363, y=w364) -> (x .and. y?=w362:bool)
      }
      frame "Störung" {
        n105 = call "Texte in VIs uebersetzen.vi"("Sprachliste"=w378, "String zum Übersetzen"="Post Test abgeschlossen") -> ("String zum Übersetzen"=w383:string)  [unwired: 9 in, 4 out]
        n106 = call "Strings und Zeitstempel verknuepfen.vi"("String 1 hinzufügen"=w383, "Eingagns String"=w381) -> ("Verknüpfter String"=w380:string)  [unwired: 9 in]
      }
      frame "Test anhalten" {
        n107 = call "FGV-Funktionstasten.vi"("Herkunft"="Drift Test", "Zustand"=Zustaende."Standby", "Aktion"=Funktionstasten-Aktion."Zustand setzen") -> ()  [unwired: 5 in, 8 out]
        n108 = call "FGV CalGas.vi"("Aktionen"=FGV_CalGas_Aktionen."Aufschaltung CalGas", "Aufschaltung CalGas"=w394) -> ()  [unwired: 5 in, 5 out]
        n109 = call "Texte in VIs uebersetzen.vi"("Sprachliste"=w404, "String zum Übersetzen"="Kein 0-Gas vorhanden. Test wurde angehalten!" ("String 1 hinzufügen")) -> ("String zum Übersetzen"=w405:string)  [unwired: 9 in, 4 out]
        n110 = call "Strings und Zeitstempel verknuepfen.vi"("String 1 hinzufügen"=w405, "Eingagns String"=w403) -> ("Verknüpfter String"=w402:string)  [unwired: 9 in]
      }
      frame "Test fortsetzen" {
        n111 = call "Texte in VIs uebersetzen.vi"("Sprachliste"=w418, "String zum Übersetzen"="Test wird fortgesetzt..." ("String 1 hinzufügen")) -> ("String zum Übersetzen"=w420:string)  [unwired: 9 in, 4 out]
        n112 = call "Strings und Zeitstempel verknuepfen.vi"("String 1 hinzufügen"=w420, "Eingagns String"=w417) -> ("Verknüpfter String"=w416:string)  [unwired: 9 in]
      }
      frame "Nachbehandlung init" {
        n113 = Select(t="Start Pre Drift Test", s=w431, f="Start Post Drift Test") -> (s? t:f=w432:string)
        n114 = call "Texte in VIs uebersetzen.vi"("Sprachliste"=w430, "String zum Übersetzen"=w432) -> ("String zum Übersetzen"=w429:string)  [unwired: 9 in, 4 out]
        n115 = call "Strings und Zeitstempel verknuepfen.vi"("String 1 hinzufügen"=w429, "Eingagns String"=w428) -> ("Verknüpfter String"=w427:string)  [unwired: 9 in]
        n116 = Get Date/Time In Seconds() -> (seconds since 1Jan1904=w441:timestamp)
      }
      frame "Nachbehandeln CG aufschalten" {
        n117 = Index Array(array=w444, index=w449) -> (element=w447:T10)
        n118 = call "FGV Drift Daten.vi"("Aktion"=Aktion_FGV_Drift_Daten."lesen") -> ("Spangaseinstellungen"=w462:T15[])  [unwired: 7 in, 7 out]
        n119 = Unbundle By Name(w447) -> ("Pretest?"=w446:bool, "Spangaseingang"=w445:i32)
        n120 = Index Array(array=w462, index=w445) -> (element=w461:T15)
        n121 = Unbundle By Name(w461) -> ("Modus"=w459:T19)
        n122 = call "Texte in VIs uebersetzen.vi"("Sprachliste"=w453, "String zum Übersetzen"="CalGas wird aufgeschalten." ("String 1 hinzufügen")) -> ("String zum Übersetzen"=w455:string)  [unwired: 9 in, 4 out]
        n123 = case shown="0, Standard" w459 {
          tunnel: w464 -> [w466 w473 w481]
          tunnel: w445 -> [w465 w472 w480]
          frame 0, Default {
            # "CG"
            n124 = call "FGV-Funktionstasten.vi"("Herkunft"="Drift Test", "Zustand"=Zustaende."Cal-Gas", "Aktion"=Funktionstasten-Aktion."Zustand setzen") -> ()  [unwired: 5 in, 8 out]
            n125 = Bundle By Name(cluster=w466, "Kalibriergas"=w465) -> (w467:T12)
            n126 = call "FGV CalGas.vi"("Aktionen"=FGV_CalGas_Aktionen."Aufschaltung CalGas", "Aufschaltung CalGas"=w467) -> ()  [unwired: 5 in, 5 out]
          }
          frame 1 {
            # "CG zu PNS"
            n127 = call "FGV-Funktionstasten.vi"("Herkunft"="Drift Test", "Zustand"=Zustaende."Cal-Gas", "Aktion"=Funktionstasten-Aktion."Zustand setzen") -> ()  [unwired: 5 in, 8 out]
            n128 = Bundle By Name(cluster=w473, "Kalibriergas"=w472, "Aufschaltpunkt"=Auswahl_Aufschaltpunkt."über PNS") -> (w474:T12)
            n129 = call "FGV CalGas.vi"("Aktionen"=FGV_CalGas_Aktionen."Aufschaltung CalGas", "Aufschaltung CalGas"=w474) -> ()  [unwired: 5 in, 5 out]
          }
          frame 2 {
            # "CG zu Externen Ventil"
            n130 = call "FGV-Funktionstasten.vi"("Herkunft"="Drift Test", "Zustand"=Zustaende."Cal-Gas", "Aktion"=Funktionstasten-Aktion."Zustand setzen") -> ("Samplepoint"=w485:u16)  [unwired: 5 in, 7 out]
            n131 = Bundle By Name(cluster=w481, "Kalibriergas"=w480, "Aufschaltpunkt"=Auswahl_Aufschaltpunkt."Entnahme") -> (w482:T12)
            n132 = call "FGV CalGas.vi"("Aktionen"=FGV_CalGas_Aktionen."Aufschaltung CalGas", "Aufschaltung CalGas"=w482) -> ()  [unwired: 5 in, 5 out]
            n133 = call "FGV Grenzwerte PNS.vi"("T90"=TRUE ("T90 lüften"), "T90 lüften"=FALSE, "Samplepoint"=w485, "Aktionen FGV Grenzwerte"=Aktionen_FGV_Grenzwerte."Anweisungscode") -> ()  [unwired: 9 in, 3 out]
          }
        }
        n134 = call "Strings und Zeitstempel verknuepfen.vi"("String 1 hinzufügen"=w455, "Eingagns String"=w452) -> ("Verknüpfter String"=w451:string)  [unwired: 9 in]
      }
      frame "Nachbehandeln CG warten" {
        n135 = call "FGV Drift Daten.vi"("Aktion"=Aktion_FGV_Drift_Daten."lesen") -> ("Drift Konfig Daten"=w513:T22)  [unwired: 7 in, 7 out]
        n136 = Unbundle By Name(w513) -> ("CG Aufschaltzeit:"=w511:dbl)
        n137 = Get Date/Time In Seconds() -> (seconds since 1Jan1904=w514:timestamp)
        n138 = Subtract(x=w514, y=w509) -> (x-y=w512:dbl)
        n139 = Greater Or Equal?(x=w512, y=w511) -> (x >= y?=w508:bool)
        n140 = Index Array(array=w495, index=w494) -> (element=w493:T10)
        n141 = Select(t=Aktion_Automatischer_Ablauf_Zustandsautomat."Nachbehandeln CG aufzeichnen", s=w508, f=w507) -> (s? t:f=w503:T1)
        n142 = case shown="True" w497 {
          tunnel: [w516 w519] -> w499
          tunnel: w498 -> [w516 w518]
          tunnel: w493 -> [_ w517]
          frame False {
          }
          frame True {
            n143 = Build Array (concatenate)(w518, w517) -> (w519:T11)
          }
        }
        n144 = Select(t=Aktion_Automatischer_Ablauf_Zustandsautomat."Störung", s=w497, f=w503) -> (s? t:f=w502:T1)
      }
      frame "Nachbehandeln CG aufzeichnen" {
        n145 = Select(t=Aktion_FGV_Drift_Daten."NB Pre Wert schreiben" ("Aktion"), s=w529, f=Aktion_FGV_Drift_Daten."NB Post Wert schreiben" ("Aktion")) -> (s? t:f=w527:T3)
        n146 = call "FGV Drift Daten.vi"("0-Gas Wert?"=FALSE, "Testnr."=w523, "Fehlercluster"=w521, "Aktion"=w527) -> ()  [unwired: 4 in, 8 out]
        n147 = Select(t="Xprespan wurde aufgezeichnet" ("String 1 hinzufügen"), s=w529, f="Xpostspan wurde aufgezeichnet" ("String 1 hinzufügen")) -> (s? t:f=w533:string)
        n148 = call "Texte in VIs uebersetzen.vi"("Sprachliste"=w534, "String zum Übersetzen"=w533) -> ("String zum Übersetzen"=w535:string)  [unwired: 9 in, 4 out]
        n149 = call "Strings und Zeitstempel verknuepfen.vi"("String 1 hinzufügen"=w535, "Eingagns String"=w532) -> ("Verknüpfter String"=w531:string)  [unwired: 9 in]
      }
    }
  }
  "Status" <- w1
  "Anzeige aktualisieren" <- w5
  "Aktion" <- w4
  "Verwendete Spangaseingänge" <- w3
  "Aktueller test" <- w2
